vi "motor_control.vi"() -> ()   [LabVIEW 2021]
uses:
  <vilib>/Analysis/Matrix/Datatypes/RealMatrix.ctl
  D:/codes/Labview/ThorLabs.MotionControl.KCube.DCServoCLI.dll
  ThorLabs.MotionControl.KCube.DCServoCLI.dll
  <vilib>/Utility/file.llb/Write Delimited Spreadsheet (DBL).vi
  D:/codes/Labview/Thorlabs.MotionControl.Controls.dll
  Thorlabs.MotionControl.Controls.dll
  <vilib>/Analysis/NI_AALBase.lvlib
  <vilib>/Analysis/Matrix/NI_Matrix.lvlib
panel:
  out "appended array":dbl[](array[numeric])
  out "output array":dbl[](array[numeric])
  in  "Delay between iterations (ms) (inner loop)":u32
  out "return count 2":u32
  out "return count":ext
  out "matrix":T1
  in  "SerialNumber":string
  in  "Start Position (mm)":dbl
  in  "Delay between iterations (ms)":u32
  in  "stop sequence":bool
  in  "End Position (mm)":dbl
  in  "step size (mm)":dbl
  out "GetPositionCounter":sgl
  in  "stop":bool
  in  "KCubeDCServoControl":refnum<k24>(container)
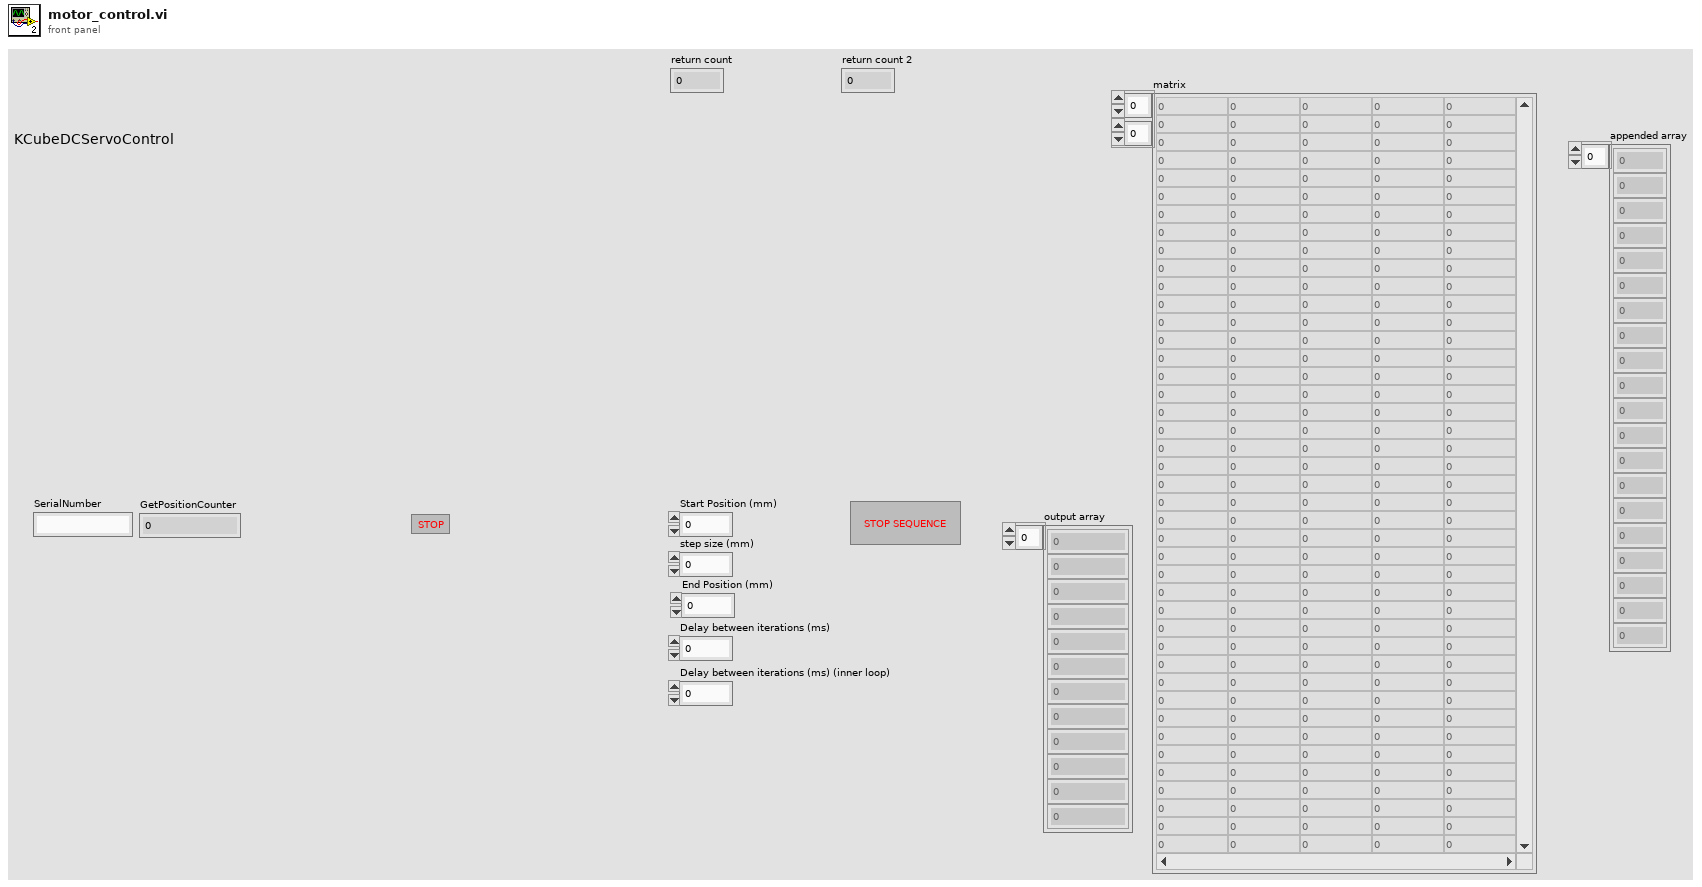
[diagram p1: front panel]
types:
  T1 = typedef "NI_Matrix.lvlib/RealMatrix.ctl" = dbl[][]
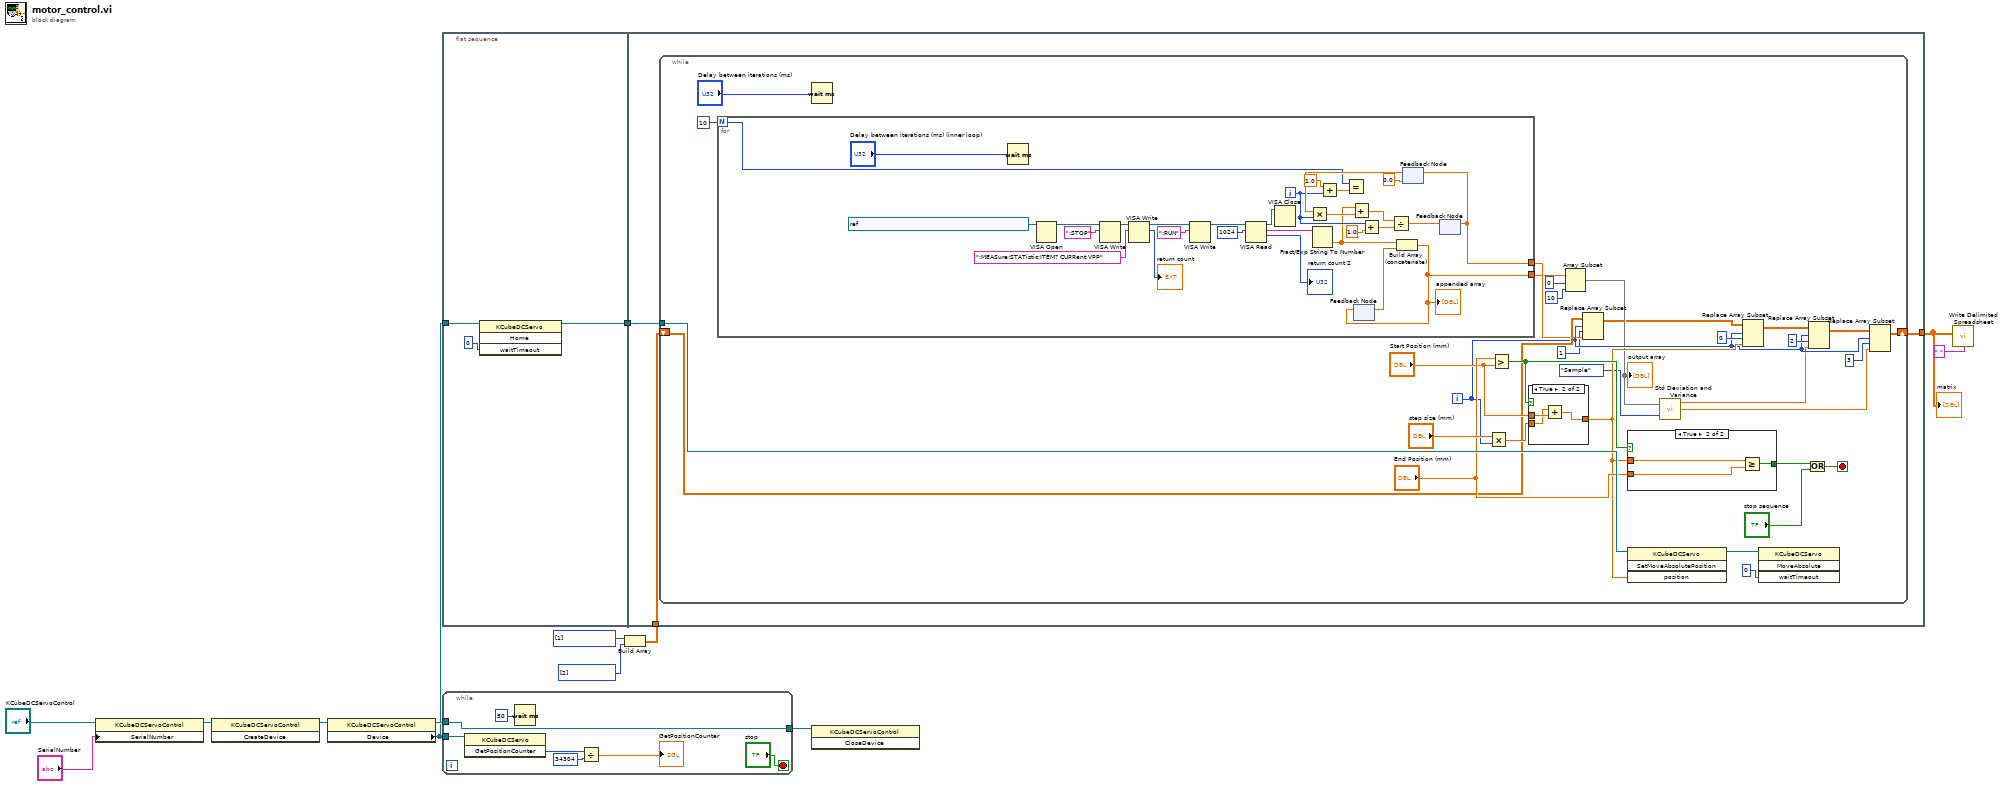
[diagram p0: block diagram]
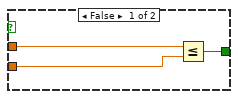
[diagram p2: hidden frame]
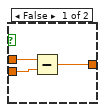
[diagram p3: hidden frame]
diagram:
  n1 = property class="KCubeDCServoControl"(reference="KCubeDCServoControl", "SerialNumber"="SerialNumber") -> (reference out=w12:refnum<k24>)  [unwired: 1 in, 1 out]
  n2 = invoke class="KCubeDCServoControl" method="CreateDevice"(reference=w12) -> (reference out=w10:refnum<k24>)  [unwired: 2 in, 2 out]
  n3 = property class="KCubeDCServoControl"(reference=w10) -> (reference out=w9:refnum<k24>, "Device"=w8:refnum<k24>)  [unwired: 1 in, 1 out]
  n4 = flat-sequence {
    tunnel: w8 -> [w15]
    tunnel: [w14] -> w6
    tunnel: w6 -> [w19]
    tunnel: w3 -> [w18]
    tunnel: [w17] -> w1
    frame #0 {
      n5 = invoke class="KCubeDCServo" method="Home"(reference=w15, "waitTimeout"=0) -> (reference out=w14:refnum<k24>)  [unwired: 2 in, 3 out]
    }
    frame #1 {
      n6 = while {
        tunnel: w19 -> [w51]
        shift-right: [w21] -> w17
        shift-left: w18 -> [w38]
        i -> [w30]
        stop <- w40 stop-if-true
        n7 = for {
          N: 10 -> [w64]
          tunnel: [w55] -> w36
          tunnel: [w60] -> w29
          i -> [w63]
          n8 = Wait (ms)(milliseconds to wait="Delay between iterations (ms) (inner loop)") -> ()  [unwired: 1 out]
          n9 = VISA Open(VISA resource name=refnum<visa-resource-name> "USB0::0x1AB1::0x0514::DS7A242600405::INSTR") -> (VISA resource name=w52:refnum<visa-resource-name>)  [unwired: 4 in, 1 out]
          n10 = VISA Write(VISA resource name=w52, write buffer=":STOP") -> (VISA resource name out=w53:refnum<visa-resource-name>)  [unwired: 1 in, 2 out]
          n11 = VISA Write(VISA resource name=w53, write buffer=":MEASure:STATistic:ITEM? CURRent,VPP") -> (VISA resource name out=w58:refnum<visa-resource-name>, return count=→"return count":u32)  [unwired: 1 in, 1 out]
          n12 = VISA Write(VISA resource name=w58, write buffer=":RUN") -> (VISA resource name out=w59:refnum<visa-resource-name>)  [unwired: 1 in, 2 out]
          n13 = VISA Read(VISA resource name=w59, byte count=u32 1024) -> (VISA resource name out=w76:refnum<visa-resource-name>, read buffer=w54:string, return count=→"return count 2":u32)  [unwired: 1 in, 1 out]
          n14 = VISA Close(VISA resource name=w76) -> ()  [unwired: 1 in, 1 out]
          n15 = Fract/Exp String To Number(string=w54) -> (number=w62:dbl)  [unwired: 3 in, 1 out]
          n16 = Add(x=1.0, y=w63) -> (x+y=w66:dbl)
          n17 = Equal?(x=w64, y=w66) -> ()  [unwired: 1 out]
          n18 = feedback #1() -> (w61:dbl[])  [unwired: 1 in]
          n19 = Add(x=w63, y=1.0) -> (x+y=w70:dbl)
          n20 = Build Array (concatenate)(w62, w61) -> (w60:dbl[])
          "appended array" <- w60
          n21 = feedback-in #1(w60) -> ()
          n22 = feedback #2(0.0) -> (w69:dbl)
          n23 = Multiply(x=w69, y=w63) -> (x*y=w73:dbl)
          n24 = Add(x=w62, y=w73) -> (x+y=w72:dbl)
          n25 = Divide(x=w72, y=w70) -> (x/y=w56:dbl)
          n26 = feedback-in #3(w56) -> ()
          n27 = feedback #3() -> (w55:dbl)  [unwired: 1 in]
          n28 = feedback-in #2(w55) -> ()
        }
        n29 = Wait (ms)(milliseconds to wait="Delay between iterations (ms)") -> ()  [unwired: 1 out]
        n30 = Multiply(x="step size (mm)", y=w30) -> (x*y=w42:dbl)
        n31 = Greater?(x="End Position (mm)", y="Start Position (mm)") -> (0:w41:bool)
        n32 = case shown="True" w41 {
          tunnel: [w87 w92] -> w35
          tunnel: "Start Position (mm)" -> [w89 w91]
          tunnel: w42 -> [w88 w90]
          frame False {
            n33 = Subtract(x=w89, y=w88) -> (x-y=w87:dbl)
          }
          frame True {
            n34 = Add(x=w90, y=w91) -> (x+y=w92:dbl)
          }
        }
        n35 = Array Subset(array=w29, index=0, length=10) -> (w25:dbl[])
        "output array" <- w25
        n36 = Replace Array Subset ("Set Matrix Elements")(array=w38, new element=w36, index (row)=w30, index (col)=1 ("disabled index (col)")) -> (w22:T1)
        n37 = case shown="True" w41 {
          tunnel: [w83 w86] -> w46
          tunnel: w35 -> [w82 w85]
          tunnel: "End Position (mm)" -> [w81 w84]
          frame False {
            n38 = Less Or Equal?(x=w82, y=w81) -> (x <= y?=w83:bool)
          }
          frame True {
            n39 = Greater Or Equal?(x=w85, y=w84) -> (x >= y?=w86:bool)
          }
        }
        n40 = invoke class="KCubeDCServo" method="SetMoveAbsolutePosition"(reference=w51, "position"=w35) -> (reference out=w49:refnum<k24>)  [unwired: 2 in, 3 out]
        n41 = call <vilib>:"Std Deviation and Variance.vi"("X"=w25, "Weighting (Sample)"=enum16{"Sample", "Population"}."Sample") -> ("mean"=w28:dbl, "standard deviation"=w27:dbl)  [unwired: 1 out]
        n42 = Replace Array Subset ("Set Matrix Elements")(array=w22, new element=w35, index (row)=w30, index (col)=0) -> (w33:T1)
        n43 = invoke class="KCubeDCServo" method="MoveAbsolute"(reference=w49, "waitTimeout"=0) -> ()  [unwired: 2 in, 4 out]
        n44 = Or(x=w46, y="stop sequence") -> (x .or. y?=w40:bool)
        n45 = Replace Array Subset ("Set Matrix Elements")(array=w33, new element=w28, index (row)=w30, index (col)=2) -> (w34:T1)
        n46 = Replace Array Subset ("Set Matrix Elements")(array=w34, new element=w27, index (row)=w30, index (col)=3) -> (w21:T1)
      }
    }
  }
  n47 = while {
    tunnel: w9 -> [w98]
    tunnel: [w98] -> w11
    tunnel: w8 -> [w94]
    stop <- "stop" stop-if-true
    n48 = invoke class="KCubeDCServo" method="GetPositionCounter"(reference=w94) -> ("GetPositionCounter"=w97:i32)  [unwired: 2 in, 2 out]
    n49 = Wait (ms)(milliseconds to wait=50) -> ()  [unwired: 1 out]
    n50 = Divide(x=w97, y=34304) -> (x/y=→"GetPositionCounter":dbl)
  }
  n51 = Build Array(u16[] [1] ("element"), u16[] [2] ("element")) -> (w3:T1)
  n52 = invoke class="KCubeDCServoControl" method="CloseDevice"(reference=w11) -> ()  [unwired: 2 in, 3 out]
  n53 = call-poly <vilib>:"Write Delimited Spreadsheet.vi"("2D data"=w1, "delimiter (\\t)"="," ("delimiter (\\t)")) -> ()  [unwired: 12 in, 2 out]
  "matrix" <- w1
